vi "Save Raw Data.vi"(1 "data":string[](array[string]), 3 "time [ms]":i64, 7 "VI-data Save":T4={"Dateipfad save data"=path "", "file ref"=refnum, "number"=0, "Period [s]"=240, "Fehler (Ausgang)"={"status"=FALSE, "code"=0, "source"=""}}) -> (8 "VI-data Save out":T4={"Dateipfad save data"=path "", "file ref"=refnum, "number"=0, "Period [s]"=240, "Fehler (Ausgang)"={"status"=FALSE, "code"=0, "source"=""}})   [LabVIEW 2010]
uses:
  VI-data Save.ctl
  control/Licor-Parameter.ctl
  Licor-Steuerung/LicorLI7000/conventions/Licor-Source.ctl
  control/Licor-Pump.ctl
  Licor-Steuerung/LicorLI7000/LicorLI7000.lvlib
panel:
  in  "Licor-parameter":T1={"CO2 ref"=392.0, "CO2 span"=402.0, "H2O ref"=0.0, "H2O span"=0.0, "Zi"=1.2, "Zt"=0.0, "Zm"=0.0, "S"=1.0, "Temp [C]"=50.0, "Pressure [hPa]"=135.0, "Licor-Sources"=["CO2A W", "CO2B W", "H2OA W", "H2OB W", "T C", "T V", "P kPa", "P V", "RH %", "CO2A um/m", "CO2B um/m", "H2OA mm/m", "H2OB mm/m"], "Licor-Pump"="Off", "Zeitstempel"=timestamp(0 s since 1904-01-01)} {"Pressure [hPa]" format="%.2g"; "Temp [C]" format="%.2f"; "CO2 ref" format="%.2f"; "CO2 span" format="%.2g"; "H2O ref" format="%.2g"; "H2O span" format="%.2g"}
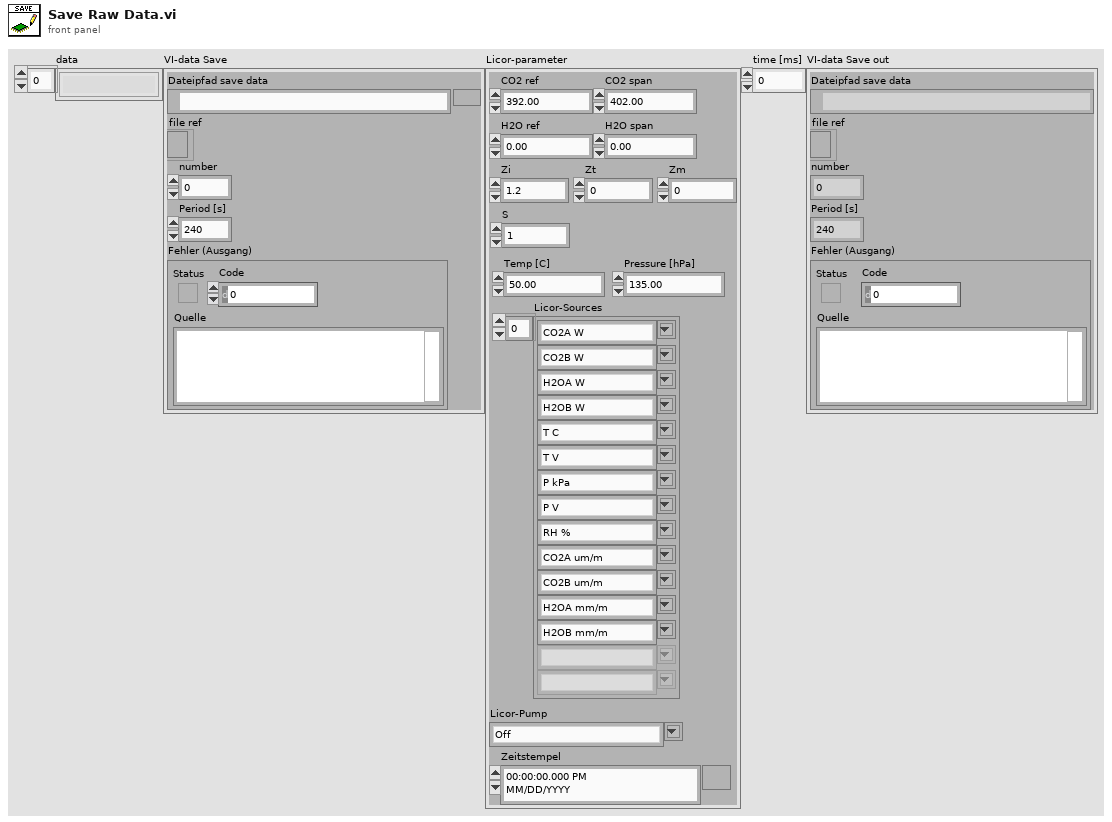
[diagram p1: front panel]
types:
  T1 = typedef "Licor-Parameter.ctl" = cluster{"CO2 ref":dbl, "CO2 span":dbl, "H2O ref":dbl, "H2O span":dbl, "Zi":dbl, "Zt":dbl, "Zm":dbl, "S":dbl, "Temp [C]":dbl, "Pressure [hPa]":dbl, "Licor-Sources":T2[], "Licor-Pump":T3, "Zeitstempel":timestamp}
  T2 = typedef "LicorLI7000.lvlib/Licor-Source.ctl" = string
  T3 = typedef "Licor-Pump.ctl" = string
  T4 = typedef "VI-data Save.ctl" = cluster{"Dateipfad save data":path, "file ref":refnum<file>, "number":i64, "Period [s]":i64, "Fehler (Ausgang)":errorcluster}
  T5 = enum16{"open", "replace", "create", "open or create", "replace or create", "replace or create with confirmation"}
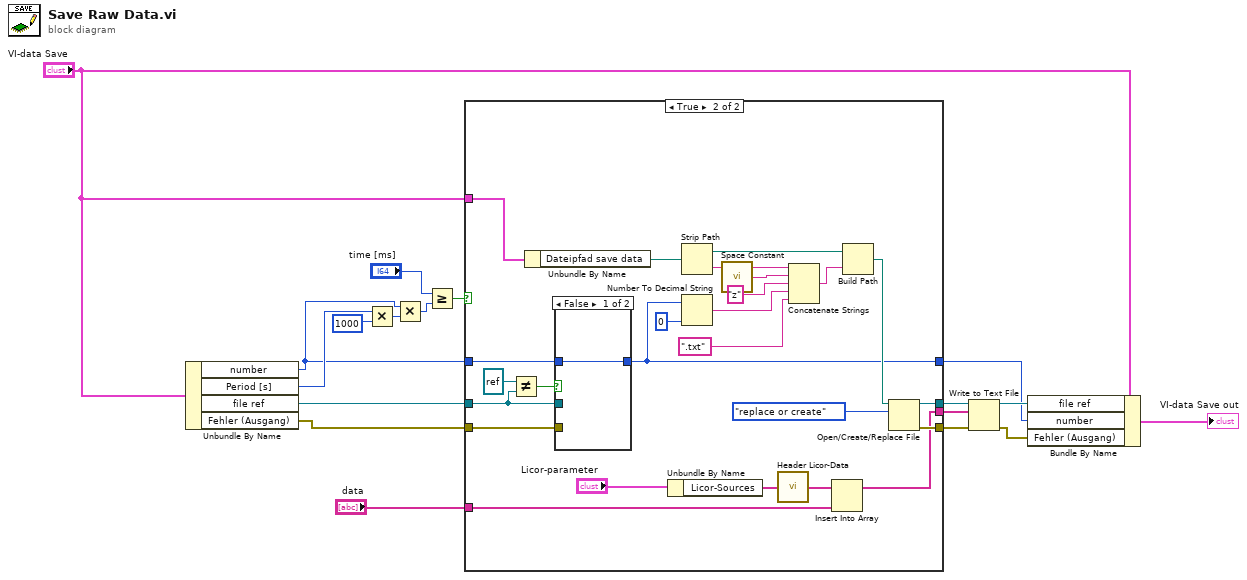
[diagram p0: block diagram]
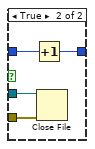
[diagram p3: hidden frame]
diagram:
  n1 = Unbundle By Name("VI-data Save") -> ("number"=w2:i64, "Period [s]"=w3:i64, "file ref"=w4:refnum<file>, "Fehler (Ausgang)"=w6:errorcluster)
  n2 = Multiply(x=w3, y=i64 1000) -> (x*y=w11:i64)
  n3 = Multiply(x=w2, y=w11) -> (x*y=w17:i64)
  n4 = Greater Or Equal?(x="time [ms]", y=w17) -> (x >= y?=w18:bool)
  n5 = case shown="True" w18 {
    tunnel: [w22 w26] -> w7
    tunnel: w2 -> [w22 w37]
    tunnel: [w21 w36] -> w15
    tunnel: w4 -> [w21 w38]
    tunnel: [w20 w45] -> w16
    tunnel: w6 -> [w20 w47]
    tunnel: "data" -> [w19 w42]
    tunnel: [w19 w41] -> w13
    tunnel: "VI-data Save" -> [_ w25]
    frame False {
    }
    frame True {
      n6 = Not Equal?(x=refnum<file> refnum ("y"), y=w38) -> (x != y?=w40:bool)
      n7 = Unbundle By Name(w25) -> ("Dateipfad save data"=w24:path)
      n8 = case shown="False" w40 {
        tunnel: w47 -> [_ w52]
        tunnel: w38 -> [_ w51]
        tunnel: w37 -> [w48 w50]
        tunnel: [w48 w49] -> w26
        frame False {
        }
        frame True {
          n9 = Increment(x=w50) -> (x+1=w49:i64)
          n10 = Close File(refnum=w51, error in=w52) -> ()  [unwired: 2 out]
        }
      }
      n11 = Unbundle By Name("Licor-parameter") -> ("Licor-Sources"=w44:T2[])
      n12 = Strip Path(path=w24) -> (stripped path=w35:path, name=w34:string)
      n13 = Number To Decimal String(number=w26, width (-)=i16 0 ("Breite (-)")) -> (decimal integer string=w30:string)
      n14 = call <vilib>:"Space Constant.vi"() -> ("String"=w32:string)
      n15 = call "Header Licor-Data.vi"("Licor-Sources"=w44) -> ("Header"=w43:string[])  [unwired: 14 in]
      n16 = Concatenate Strings(w34, w32, "z", w30, ".txt") -> (w28:string)
      n17 = Insert Into Array(array=w43, new element=w42) -> (w41:string[])  [unwired: 1 in]
      n18 = Build Path(base path=w35, name or relative path=w28) -> (appended path=w27:path)
      n19 = Open/Create/Replace File(file path (use dialog)=w27, operation (0:open)=T5."replace or create" ("Operation (0:Öffnen)")) -> (refnum out=w36:refnum<file>, error out=w45:errorcluster)  [unwired: 4 in, 1 out]
    }
  }
  n20 = Write to Text File(file (use dialog)=w15, text=w13, error in=w16) -> (refnum out=w9:refnum<file>, error out=w8:errorcluster)  [unwired: 1 in, 1 out]
  n21 = Bundle By Name(cluster="VI-data Save", "file ref"=w9, "number"=w7, "Fehler (Ausgang)"=w8) -> (→"VI-data Save out":T4)
